vi "TCP Loop.vi"(8 "error in":errorcluster, 10 "Queues":T1, 11 "Notifiers":T2) -> (0 "error out":errorcluster)   [LabVIEW 2014, in "TCP.lvlib"]
uses:
  TCP.lvlib
  support/Message Queue/Message Queue.lvlib
  <vilib>/ErrorRing/Error Ring.xnode
  TypeDefs/TCP Data.ctl
  <vilib>/Utility/error.llb/Error Cluster From Error Code.vi
  Support/Global names.vi
  SubVIs/TCP global names.vi
  Support/Message Queue/Message Cluster.ctl
  Support/Notifiers/Notifiers.ctl
  Support/Notifiers/Notifiers.lvlib
  Support/Message Queue/All Message Queues.ctl
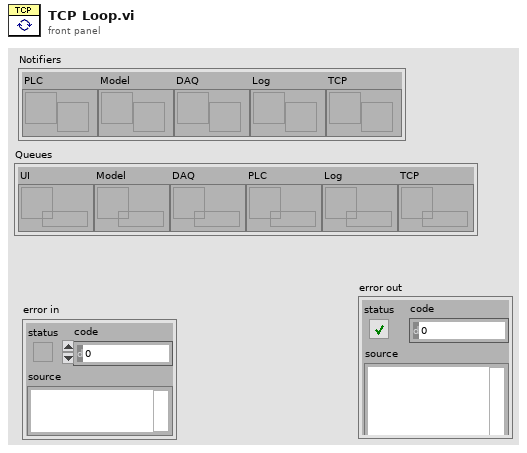
[diagram p1: front panel]
types:
  T1 = typedef "Message Queue.lvlib/All Message Queues.ctl" = cluster{"UI":refnum<queue>, "Model":refnum<queue>, "DAQ":refnum<queue>, "PLC":refnum<queue>, "Log":refnum<queue>, "TCP":refnum<queue>}
  T2 = typedef "Notifiers.lvlib/Notifiers.ctl" = cluster{"PLC":refnum<notifier>, "Model":refnum<notifier>, "DAQ":refnum<notifier>, "Log":refnum<notifier>, "TCP":refnum<notifier>}
  T3 = typedef "TCP.lvlib/TCP Data.ctl" = cluster{"Type":enum16{"Server", "Client"}, "IP":string, "Port":u16, "connection ID":refnum<k5>, "Connected?":bool, "Data":string}
  T4 = enum16{"Standard", "Buffered", "CRLF", "Immediate"}
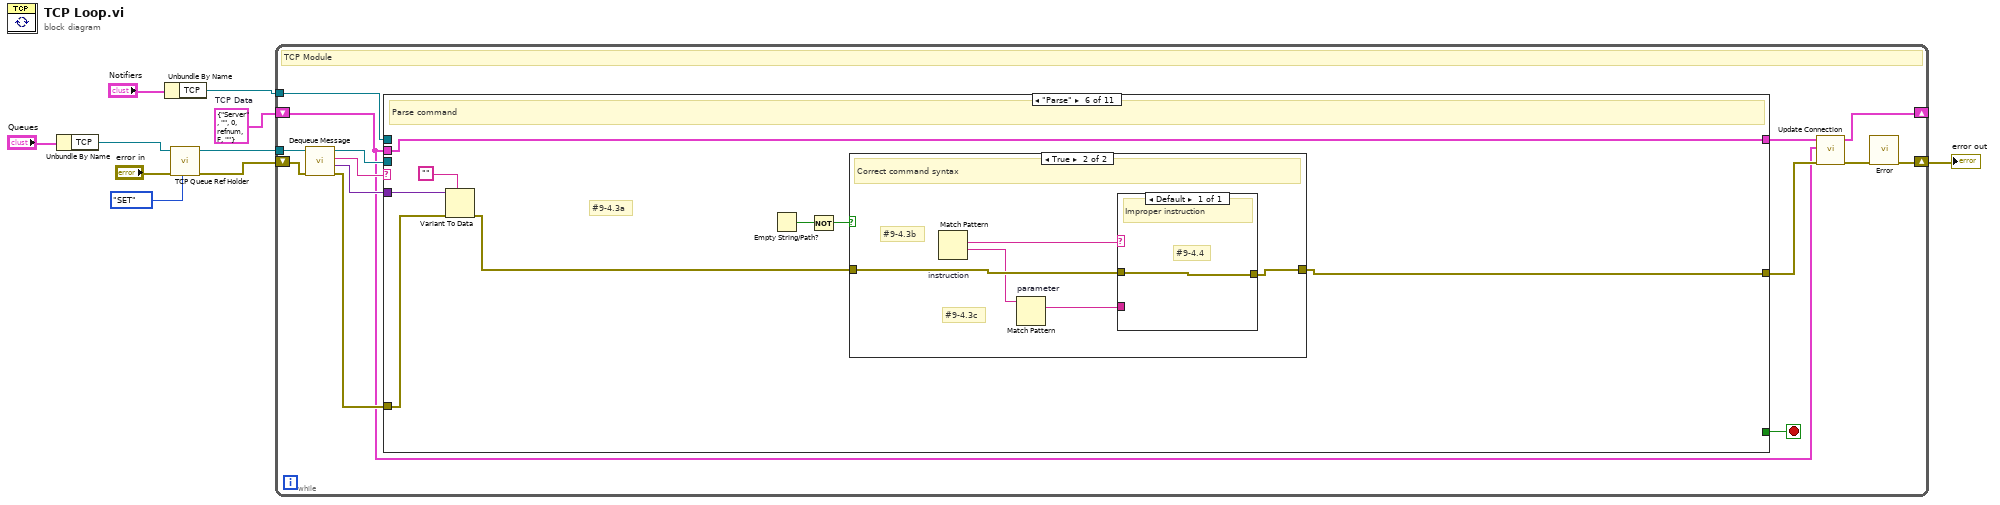
[diagram p0: block diagram]
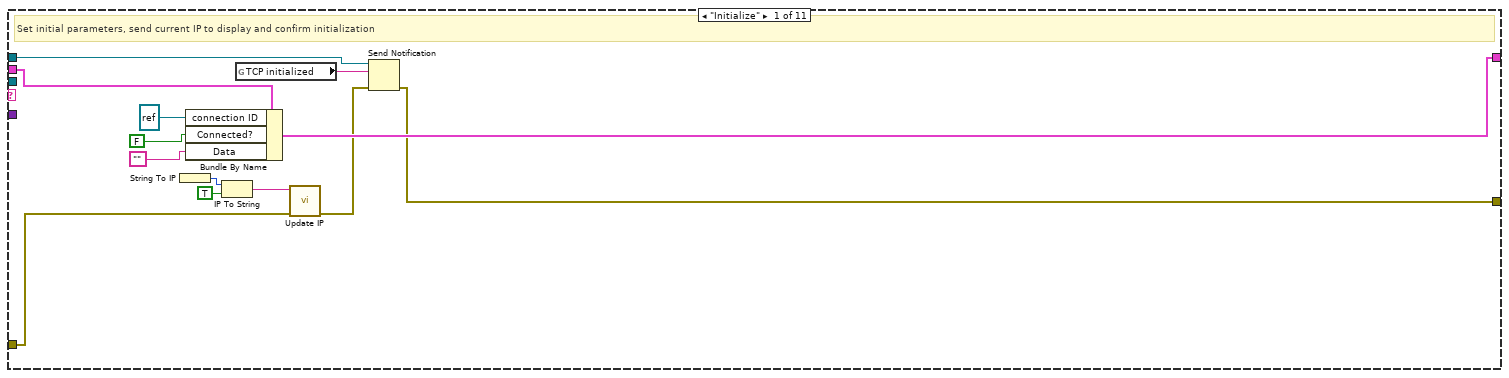
[diagram p2: hidden frame]
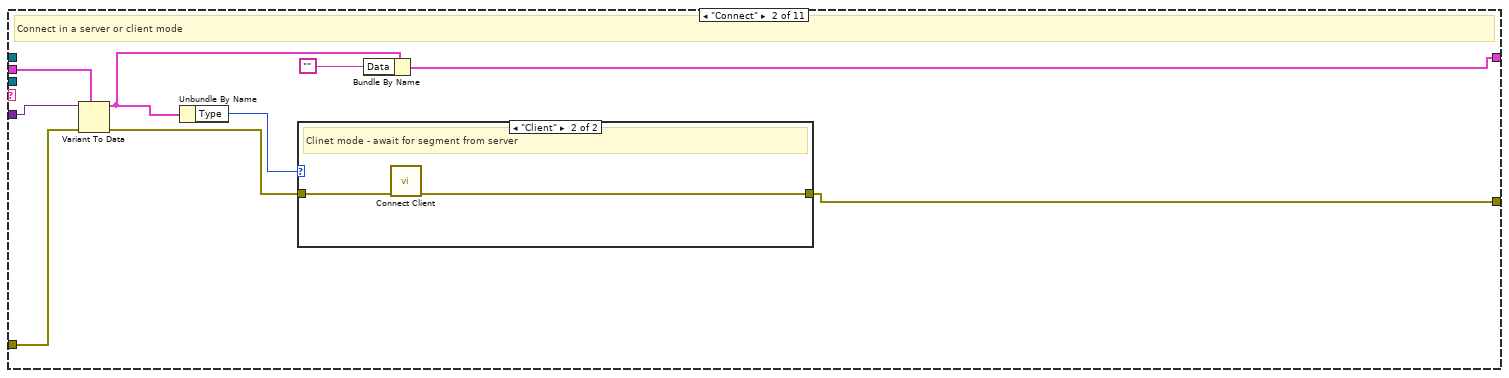
[diagram p3: hidden frame]
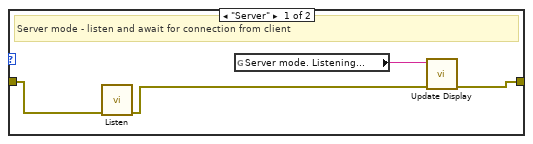
[diagram p4: hidden frame]
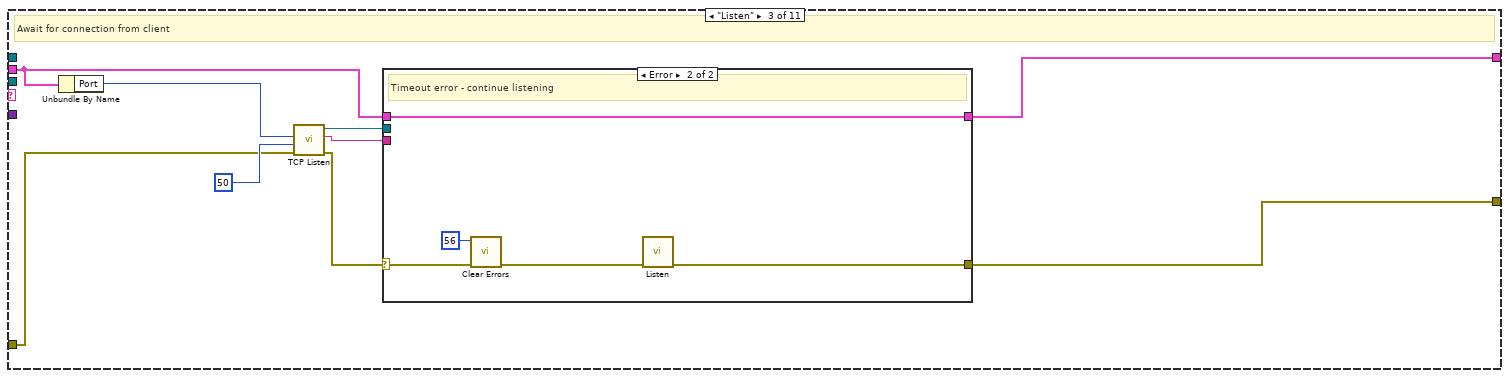
[diagram p5: hidden frame]
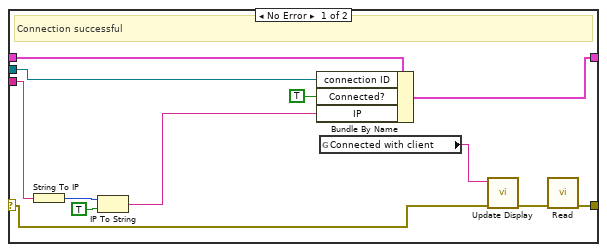
[diagram p6: hidden frame]
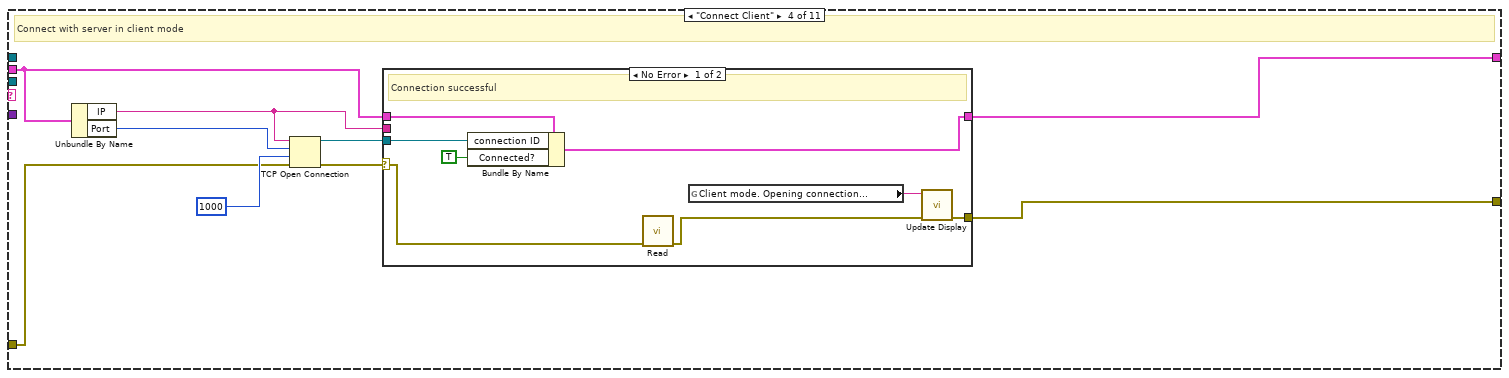
[diagram p7: hidden frame]
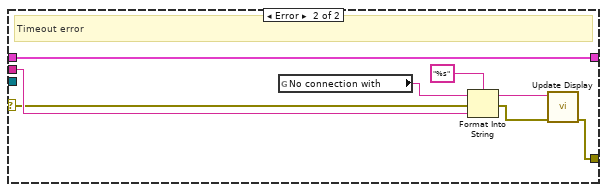
[diagram p8: hidden frame]
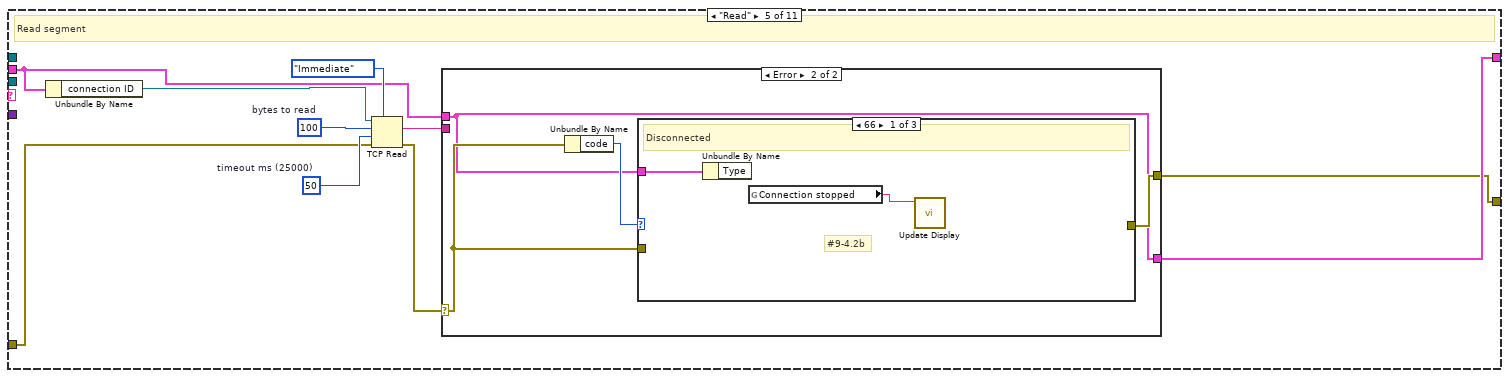
[diagram p9: hidden frame]
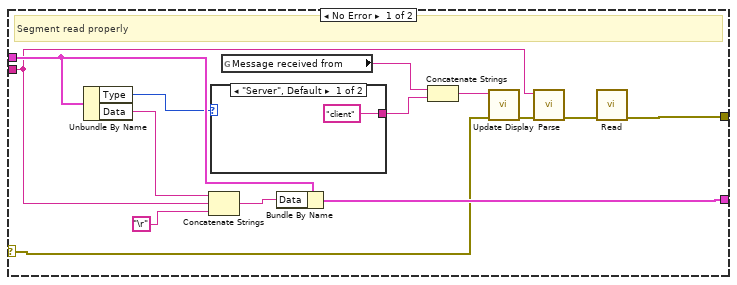
[diagram p10: hidden frame]
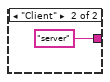
[diagram p11: hidden frame]
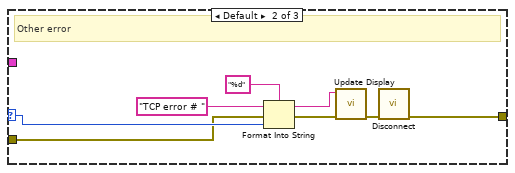
[diagram p12: hidden frame]
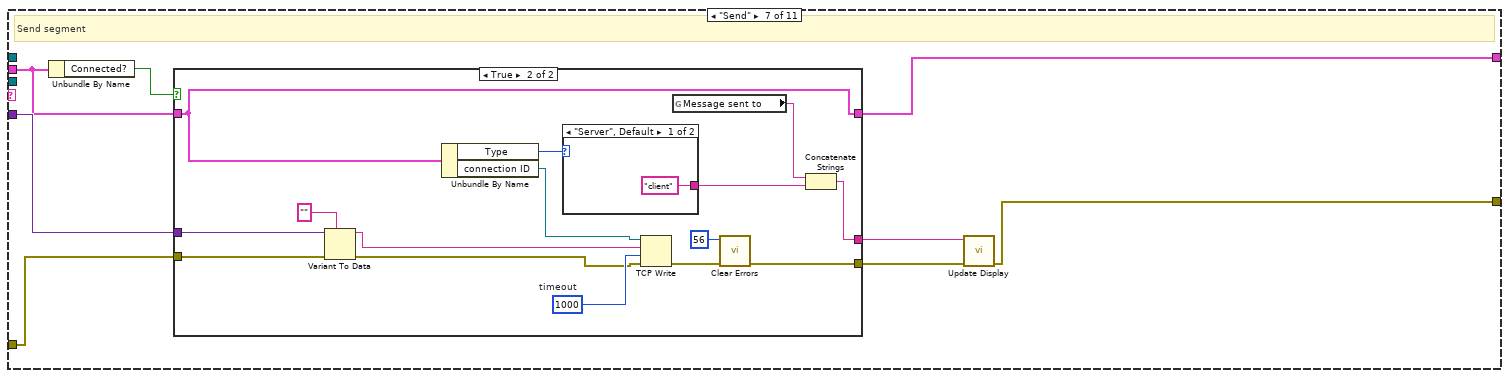
[diagram p15: hidden frame]
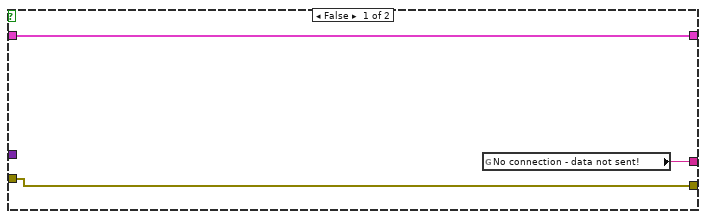
[diagram p16: hidden frame]
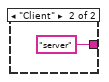
[diagram p17: hidden frame]
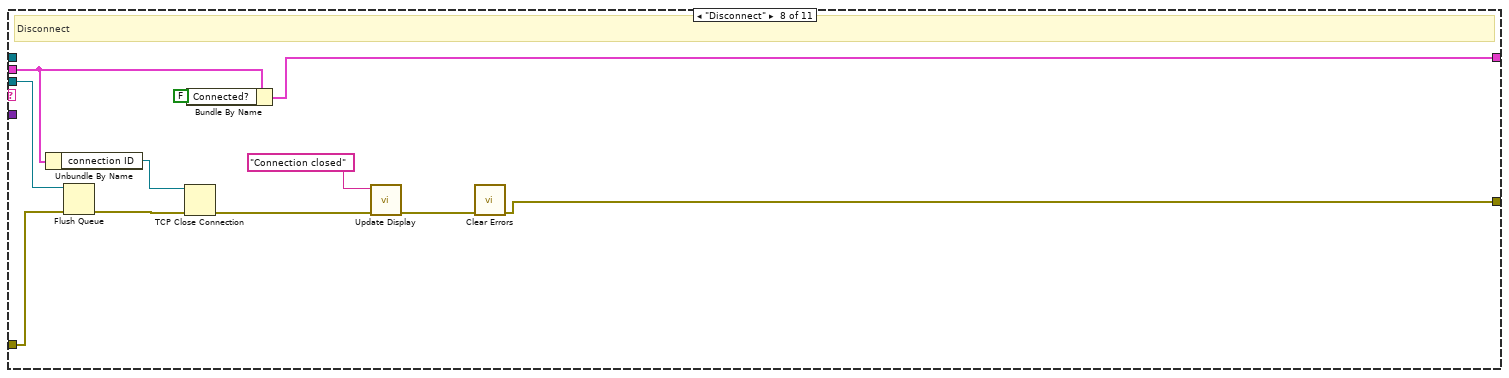
[diagram p18: hidden frame]
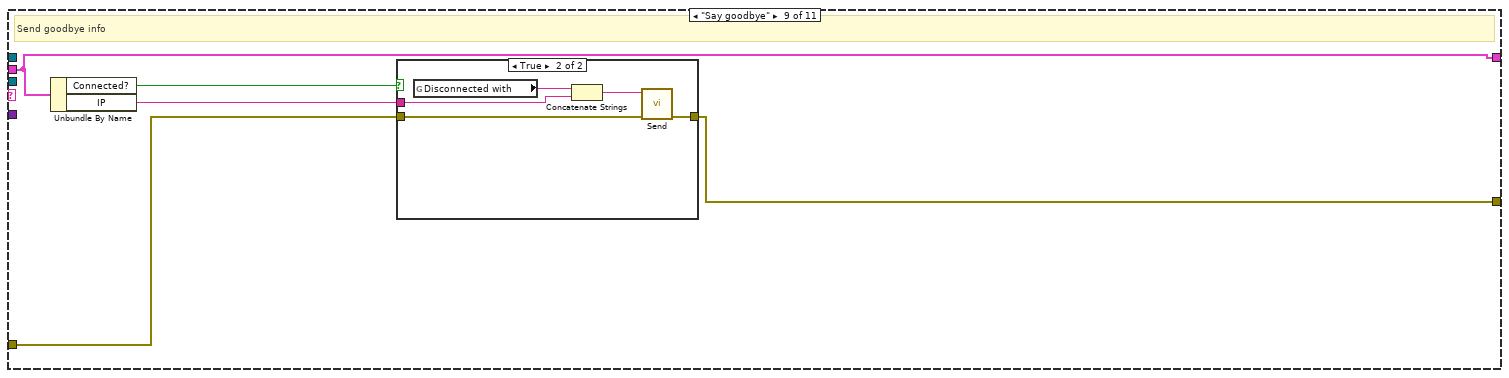
[diagram p19: hidden frame]
diagram:
  w10 = T3 {"Type"=enum."Server", "IP"="", "Port"=0, "connection ID"=refnum, "Connected?"=FALSE, "Data"=""}  # TCP Data
  n1 = Unbundle By Name("Queues") -> ("TCP"=w3:refnum<queue>)
  n2 = Unbundle By Name("Notifiers") -> ("TCP"=w4:refnum<notifier>)
  n3 = call "TCP Queue Ref Holder.vi"("Action"=enum16{"GET", "SET"}."SET", "error in"="error in", "Message Queue In"=w3) -> ("error out"=w7:errorcluster, "Input Message Queue"=w9:refnum<queue>)  [unwired: 7 in]
  n4 = while {
    tunnel: w9 -> [w24]
    tunnel: w4 -> [w19]
    shift-right: [w14] -> _
    shift-left: w10 -> [w11]
    shift-right: [w13] -> w1
    shift-left: w7 -> [w23]
    stop <- w20 stop-if-true
    # "TCP Module"
    n5 = call "Dequeue Message.vi"("error in (no error)"=w23, "Message Queue"=w24) -> ("error out"=w21:errorcluster, "Message Data"=w18:variant, "Message"=w22:string, "dup Message Queue"=w12:refnum<queue>)  [unwired: 6 in]
    n6 = case shown="\"Parse\"" w22 {
      selector: w22 -> [_ _ _ _ _ _ _ _ _ _ w222]
      tunnel: w21 -> [w28 w46 w54 w79 w104 w149 w166 w192 w201 w219 _]
      tunnel: [w30 w45 w58 w82 w105 w146 w160 w188 w202 w216 w221] -> w17
      tunnel: [_ _ _ _ _ _ _ _ _ TRUE _] -> w20
      tunnel: w19 -> [w29 _ _ _ _ _ _ _ _ w214 _]
      tunnel: w11 -> [w37 w39 w56 w84 w107 w148 w163 w196 w200 w212 w220]
      tunnel: [w36 w43 w55 w83 w106 w148 w164 w197 w200 w211 w220] -> w15
      tunnel: w18 -> [_ w44 _ _ _ w151 w165 _ _ _ _]
      tunnel: w12 -> [_ _ _ _ _ _ _ w187 _ w209 _]
      frame "Initialize" {
        # "Set initial parameters, send current IP to display and confirm initialization"
        n7 = String To IP() -> (0:w31:u32)  [unwired: 1 in]
        n8 = Bundle By Name(cluster=w37, "connection ID"=refnum<k5> refnum, "Connected?"=FALSE, "Data"="") -> (w36:T3)
        n9 = IP To String(1:TRUE ("dot notation? (F)"), 2:w31) -> (0:w25:string)
        n10 = global read "Global names.vi" "TCP initialized"() -> (w26:string)
        n11 = call "Update IP.vi"("error in"=w28, "Message string"=w25) -> ("error out"=w27:errorcluster)  [unwired: 9 in]
        n12 = Send Notification(notification=w26, notifier=w29, error in (no error)=w27) -> (error out=w30:errorcluster)  [unwired: 1 out]
      }
      frame "Connect" {
        # "Connect in a server or client mode"
        n13 = Variant To Data(error in=w46, type=w39, Variant=w44) -> (data=w38:T3, error out=w42:errorcluster)
        n14 = Unbundle By Name(w38) -> ("Type"=w40:enum16{"Server", "Client"})
        n15 = case shown="\"Client\"" w40 {
          tunnel: w42 -> [w50 w52]
          tunnel: [w48 w51] -> w45
          frame "Server" {
            # "Server mode - listen and await for connection from client"
            n16 = call "Listen.vi"("error in"=w50) -> ("error out"=w49:errorcluster)  [unwired: 10 in]
            n17 = global read "TCP global names.vi" "Server mode. Listening..."() -> (w47:string)
            n18 = call "Update Display.vi"("error in"=w49, "Message string"=w47) -> ("error out"=w48:errorcluster)  [unwired: 9 in]
          }
          frame "Client" {
            # "Clinet mode - await for segment from server"
            n19 = call "Connect Client.vi"("error in"=w52) -> ("error out"=w51:errorcluster)  [unwired: 10 in]
          }
        }
        n20 = Bundle By Name(cluster=w38, "Data"="") -> (w43:T3)
      }
      frame "Listen" {
        # "Await for connection from client"
        n21 = Unbundle By Name(w56) -> ("Port"=w61:u16)
        n22 = call <vilib>:"TCP Listen.vi"("error in (no error)"=w54, "timeout ms (wait forever: -1)"=50, "port"=w61) -> ("error out"=w59:errorcluster, "remote address"=w53:string, "connection ID"=w57:refnum<k5>)  [unwired: 4 in, 2 out]
        n23 = case shown="Error" w59 {
          selector: w59 -> [w62 w74]
          tunnel: [w68 w76] -> w58
          tunnel: w57 -> [w72 _]
          tunnel: w56 -> [w73 w77]
          tunnel: [w70 w77] -> w55
          tunnel: w53 -> [w66 _]
          frame No Error {
            # "Connection successful"
            n24 = String To IP(1:w66) -> (0:w65:u32)
            n25 = IP To String(1:TRUE ("dot notation? (F)"), 2:w65) -> (0:w63:string)
            n26 = Bundle By Name(cluster=w73, "connection ID"=w72, "Connected?"=TRUE, "IP"=w63) -> (w70:T3)
            n27 = global read "TCP global names.vi" "Connected with client"() -> (w67:string)
            n28 = call "Update Display.vi"("error in"=w62, "Message string"=w67) -> ("error out"=w69:errorcluster)  [unwired: 9 in]
            n29 = call "Read.vi"("error in"=w69) -> ("error out"=w68:errorcluster)  [unwired: 10 in]
          }
          frame Error {
            # "Timeout error - continue listening"
            n30 = call <vilib>:"Clear Errors.vi"("error in (no error)"=w74, "specific error code to clear (0: all)"=56) -> ("error out"=w75:errorcluster)  [unwired: 4 in, 1 out]
            n31 = call "Listen.vi"("error in"=w75) -> ("error out"=w76:errorcluster)  [unwired: 10 in]
          }
        }
      }
      frame "Connect Client" {
        # "Connect with server in client mode"
        n32 = Unbundle By Name(w84) -> ("IP"=w81:string, "Port"=w80:u16)
        n33 = TCP Open Connection(address=w81, remote port or service name=w80, timeout ms (60000)=1000, error in (no error)=w79) -> (connection ID=w85:refnum<k5>, error out=w86:errorcluster)  [unwired: 1 in]
        n34 = case shown="No Error" w86 {
          selector: w86 -> [w89 w98]
          tunnel: [w92 w97] -> w83
          tunnel: w85 -> [w94 _]
          tunnel: w84 -> [w95 w97]
          tunnel: [w91 w100] -> w82
          tunnel: w81 -> [_ w102]
          frame No Error {
            # "Connection successful"
            n35 = Bundle By Name(cluster=w95, "connection ID"=w94, "Connected?"=TRUE) -> (w92:T3)
            n36 = call "Read.vi"("error in"=w89) -> ("error out"=w90:errorcluster)  [unwired: 10 in]
            n37 = global read "TCP global names.vi" "Client mode. Opening connection..."() -> (w88:string)
            n38 = call "Update Display.vi"("error in"=w90, "Message string"=w88) -> ("error out"=w91:errorcluster)  [unwired: 9 in]
          }
          frame Error {
            # "Timeout error"
            n39 = global read "TCP global names.vi" "No connection with"() -> (w96:string)
            n40 = Format Into String(format string="%s", initial string=w96, error in=w98, w102) -> (resulting string=w99:string, error out=w101:errorcluster)
            n41 = call "Update Display.vi"("error in"=w101, "Message string"=w99) -> ("error out"=w100:errorcluster)  [unwired: 9 in]
          }
        }
      }
      frame "Read" {
        w111 = 50  # timeout ms (25000)
        w112 = 100  # bytes to read
        # "Read segment"
        n42 = Unbundle By Name(w107) -> ("connection ID"=w113:refnum<k5>)
        n43 = TCP Read(connection ID=w113, bytes to read=w112, error in (no error)=w104, 7:T4."Immediate" ("mode (standard)"), 9:w111) -> (data out=w108:string, error out=w109:errorcluster)  [unwired: 1 out]
        n44 = case shown="Error" w109 {
          selector: w109 -> [w117 w132]
          tunnel: [w127 w130] -> w106
          tunnel: w108 -> [w121 _]
          tunnel: w107 -> [w126 w130]
          tunnel: [w118 w131] -> w105
          frame No Error {
            # "Segment read properly"
            n45 = Unbundle By Name(w126) -> ("Type"=w124:enum16{"Server", "Client"}, "Data"=w115:string)
            n46 = Concatenate Strings(w115, w121, "\r") -> (w125:string)
            n47 = case shown="\"Server\", Default" w124 {
              tunnel: ["client" ("Message") "server" ("f")] -> w123
              frame "Server", Default {
              }
              frame "Client" {
              }
            }
            n48 = global read "TCP global names.vi" "Message received from"() -> (w116:string)
            n49 = Bundle By Name(cluster=w126, "Data"=w125) -> (w127:T3)
            n50 = Concatenate Strings(w116, w123) -> (w120:string)
            n51 = call "Update Display.vi"("error in"=w117, "Message string"=w120) -> ("error out"=w122:errorcluster)  [unwired: 9 in]
            n52 = call "Parse.vi"("error in"=w122, "String"=w121) -> ("error out"=w119:errorcluster)  [unwired: 9 in]
            n53 = call "Read.vi"("error in"=w119) -> ("error out"=w118:errorcluster)  [unwired: 10 in]
          }
          frame Error {
            n54 = Unbundle By Name(w132) -> ("code"=w133:i32)
            n55 = case shown="66" w133 {
              selector: w133 -> [_ w141 _]
              tunnel: w132 -> [_ w136 _]
              tunnel: w130 -> [w135 _ _]
              tunnel: [_ w137 _] -> w131
              frame 66 {
                # "#9-4.2b"
                # "Disconnected"
                n56 = Unbundle By Name(w135) -> ()  [unwired: 1 out]
                n57 = global read "TCP global names.vi" "Connection stopped"() -> (w134:string)
                n58 = call "Update Display.vi"("Message string"=w134) -> ()  [unwired: 10 in, 1 out]
              }
              frame Default {
                # "Other error"
                n59 = Format Into String(format string="%d", initial string="TCP error # " ("Message"), error in=w136, w141) -> (resulting string=w139:string, error out=w140:errorcluster)
                n60 = call "Update Display.vi"("error in"=w140, "Message string"=w139) -> ("error out"=w138:errorcluster)  [unwired: 9 in]
                n61 = call "Disconnect.vi"("error in"=w138) -> ("error out"=w137:errorcluster)  [unwired: 10 in]
              }
              frame 56 {
                # "#9-4.2a"
                # "Timeout"
              }
            }
          }
        }
      }
      frame "Parse" {
        # "#9-4.3a"
        # "Parse command"
        n62 = Variant To Data(error in=w149, type="", Variant=w151) -> (error out=w147:errorcluster)  [unwired: 1 out]
        n63 = Empty String/Path?() -> (empty?=w145:bool)  [unwired: 1 in]
        n64 = Not(x=w145) -> (.not. x?=w144:bool)
        n65 = case shown="True" w144 {
          tunnel: w147 -> [w152 w157]
          tunnel: [w152 w156] -> w146
          frame False {
            # "Incorrect command"
          }
          frame True {
            # "#9-4.3c"
            # "#9-4.3b"
            # "Correct command syntax"
            n66 = Match Pattern "instruction"() -> (match substring=w155:string, after substring=w154:string)  [unwired: 3 in, 2 out]
            n67 = Match Pattern "parameter"(string=w154) -> (match substring=w153:string)  [unwired: 2 in, 3 out]
            n68 = case shown="Default" w155 {
              tunnel: w157 -> [w158]
              tunnel: [w158] -> w156
              tunnel: w153 -> [_]
              frame Default {
                # "#9-4.4"
                # "Improper instruction"
              }
            }
          }
        }
      }
      frame "Send" {
        # "Send segment"
        n69 = Unbundle By Name(w163) -> ("Connected?"=w162:bool)
        n70 = case shown="True" w162 {
          tunnel: w166 -> [w169 w184]
          tunnel: w165 -> [_ w183]
          tunnel: w163 -> [w168 w173]
          tunnel: [w168 w173] -> w164
          tunnel: [w167 w176] -> w159
          tunnel: [w169 w174] -> w161
          frame False {
            n71 = global read "TCP global names.vi" "No connection - data not sent!"() -> (w167:string)
          }
          frame True {
            w179 = 1000  # timeout
            n72 = Variant To Data(error in=w184, type="", Variant=w183) -> (data=w170:string, error out=w175:errorcluster)
            n73 = Unbundle By Name(w173) -> ("Type"=w178:enum16{"Server", "Client"}, "connection ID"=w171:refnum<k5>)
            n74 = case shown="\"Server\", Default" w178 {
              tunnel: ["client" ("Message") "server" ("f")] -> w177
              frame "Server", Default {
              }
              frame "Client" {
              }
            }
            n75 = TCP Write(connection ID=w171, data in=w170, error in (no error)=w175, 9:w179) -> (error out=w181:errorcluster)  [unwired: 2 out]
            n76 = global read "TCP global names.vi" "Message sent to"() -> (w172:string)
            n77 = call <vilib>:"Clear Errors.vi"("error in (no error)"=w181, "specific error code to clear (0: all)"=56) -> ("error out"=w174:errorcluster)  [unwired: 4 in, 1 out]
            n78 = Concatenate Strings(w172, w177) -> (w176:string)
          }
        }
        n79 = call "Update Display.vi"("error in"=w161, "Message string"=w159) -> ("error out"=w160:errorcluster)  [unwired: 9 in]
      }
      frame "Disconnect" {
        # "Disconnect"
        n80 = Unbundle By Name(w196) -> ("connection ID"=w195:refnum<k5>)
        n81 = Flush Queue(queue=w187, error in (no error)=w192) -> (error out=w191:errorcluster)  [unwired: 2 out]
        n82 = TCP Close Connection(connection ID=w195, error in (no error)=w191) -> (error out=w190:errorcluster)  [unwired: 1 in, 1 out]
        n83 = Bundle By Name(cluster=w196, "Connected?"=FALSE) -> (w197:T3)
        n84 = call "Update Display.vi"("error in"=w190, "Message string"="Connection closed" ("Message")) -> ("error out"=w189:errorcluster)  [unwired: 9 in]
        n85 = call <vilib>:"Clear Errors.vi"("error in (no error)"=w189) -> ("error out"=w188:errorcluster)  [unwired: 5 in, 1 out]
      }
      frame "Say goodbye" {
        # "Send goodbye info"
        n86 = Unbundle By Name(w200) -> ("Connected?"=w198:bool, "IP"=w199:string)
        n87 = case shown="True" w198 {
          tunnel: [w203 w208] -> w202
          tunnel: w201 -> [w203 w207]
          tunnel: w199 -> [_ w206]
          frame False {
          }
          frame True {
            n88 = global read "TCP global names.vi" "Disconnected with"() -> (w204:string)
            n89 = Concatenate Strings(w204, w206) -> (w205:string)
            n90 = call "Send.vi"("error in"=w207, "Data"=w205) -> ("error out"=w208:errorcluster)  [unwired: 9 in]
          }
        }
      }
      frame "Exit" {
        # "Release queue, send exit notification and quit TCP loop"
        n91 = Bundle By Name(cluster=w212, "Connected?"=FALSE) -> (w211:T3)
        n92 = Release Queue(queue=w209, force destroy? (F)=TRUE, error in (no error)=w219) -> (error out=w217:errorcluster)  [unwired: 2 out]
        n93 = global read "Global names.vi" "TCP exit"() -> (w210:string)
        n94 = Send Notification(notification=w210, notifier=w214, error in (no error)=w217) -> (error out=w216:errorcluster)  [unwired: 1 out]
      }
      frame Default {
        # "Incorrect message"
        n95 = xnode "Error Ring"("parameter 0"=w222) -> ("error out"=w221:errorcluster)
      }
    }
    n96 = call "Update Connection.vi"("error in (no error)"=w17, "TCP Data before update"=w11, "TCP Data after update"=w15) -> ("error out"=w16:errorcluster, "TCP Data after update out"=w14:T3)  [unwired: 7 in]
    n97 = call "Error.vi"("error in"=w16) -> ("error out"=w13:errorcluster)  [unwired: 10 in]
  }
  "error out" <- w1
